vi "NMRglobal.vi"() -> ()   [LabVIEW 2013]
uses:
  <vilib>/Analysis/NI_AALBase.lvlib
panel:
  out "NMR Ave Graph":cluster{dbl, "Step Width (MHz)":dbl, dbl[][]}(graph)={224.69, "Step Width (MHz)"=0.002, [[-0.0025585333333335973, -0.0025785333333285033, -0.0021201333333384976, -0.0024833333333335096, -0.002168133333328727, -7.453333333811774e-05, -0.0018025333333334345, -0.003952133333328963, -0.0024233333333377447, -0.003016133333333376, -0.0035305333333292195, -0.00456653333333739, -0.004924133333333334, -0.007103333333329486, -0.0072041333333370495, -0.0031265333333333066, -0.0019705333333297687, -0.0005361333333367225, -0.001523333333333292, -0.0008321333333300675, 0.0001374666666635896, -0.00021453333333329298, 0.0004118666666696188, -0.00028333333333611444, -0.0004001333333333079, 0.004161466666669293, 0.001801466666664166, 0.0007198666666666612, 0.00171666666666895, -0.0009081333333355671, -0.0017545333333333839, -0.00012253333333140683, -0.0015121333333353152, -0.0021233333333334436, -0.0002561333333317787, -0.0012105333333350776, -0.0008865333333335181, -0.001584133333332165, -0.001903333333334855, -0.0022441333333336074, 9.346666666743345e-05, -0.0007905333333346475, 0.0017038666666662878, 0.005276666666667018, 0.007927866666665546, 0.008557466666666168, 0.012365466666666587, 0.02055186666666572, 0.028516666666666034, 0.03605986666666614, 0.041481466666665884, 0.04718146666666588, 0.045159866666665674, 0.04401666666666603, 0.03575186666666572, 0.028465466666665204, 0.02345746666666617, 0.020327866666665542, 0.017976666666664715, 0.014003866666666288, 0.013809466666665353, 0.014493466666664212, 0.014755866666666392, 0.008196666666665145, 0.009715866666667836, 0.008813466666666483, 0.009389466666664922, 0.008543866666668221, 0.0073766666666665575, 0.005687866666664685, 0.0066774666666685936, 0.005945466666666617, 0.0047918666666644325, 0.005516666666668951, 0.0014198666666666612, 0.0012014666666641661, 0.003161466666669293, 0.0032998666666666913, 0.00011666666666388487, -0.0009881333333303806, -0.0022145333333332923, 0.0013374666666635892, 0.00046786666666993155, 0.0008766666666667075, -0.0018361333333367235, -0.0004705333333297673, -0.0003265333333333061, -0.0020041333333370493, -0.001903333333329486, -0.0008241333333333347, -0.00236653333333739, -0.00313053333332922, 0.000583866666666625, 0.0019766666666622564, 0.002347866666671036, 0.004297466666666567, 0.005125466666661882, 0.004031866666671274, 0.006916666666666493, 0.0074798666666615, 0.006521466666671498], [-0.004151555000000268, -0.0032346549999951674, -0.0030565550000051585, -0.0030515550000001757, -0.003032154999995392, -0.0029464550000047837, -0.0028670550000001005, -0.002839254999995635, -0.0028472550000044083, -0.0028393550000000403, -0.0026902549999958864, -0.002623055000004056, -0.0025824550000000004, -0.002625554999996152, -0.002628855000003716, -0.002497254999999975, -0.002488654999996437, -0.002326755000003392, -0.002277254999999956, -0.0021894549999967312, -0.002116355000003079, -0.0020416549999999595, -0.002037954999997048, -0.0019417550000027821, -0.0018279549999999749, -0.0017424549999973742, -0.0016252550000024997, -0.0014985550000000051, -0.0013201549999977155, -0.0011361550000022333, -0.0010181550000000496, -0.0008573549999980733, -0.0006557550000019807, -0.00040805500000011004, -0.00021615499999844492, -2.1755000001744238e-05, 0.00028584499999981494, 0.0006856450000011681, 0.0012884449999984791, 0.0017766449999997254, 0.002533845000000767, 0.003499044999998682, 0.004639044999999614, 0.006053645000000351, 0.007976744999998881, 0.010652944999999504, 0.014275344999999917, 0.019335044999999062, 0.025848744999999354, 0.03369944499999943, 0.04110654499999926, 0.04502774499999923, 0.04310974499999907, 0.03670224499999938, 0.029105044999999042, 0.022443844999998505, 0.017336244999999504, 0.013608844999998863, 0.010775244999998053, 0.008735444999999623, 0.007194644999998683, 0.006035844999997543, 0.005142344999999731, 0.004461544999998471, 0.003983745000001169, 0.0036107449999998173, 0.0032414449999982517, 0.0030450450000015557, 0.0027286449999998916, 0.002523044999998015, 0.0023226450000019255, 0.0022273449999999527, 0.0021633449999977654, 0.002135445000002284, 0.002108244999999996, 0.0020771449999975, 0.0020462450000026285, 0.002019145000000028, 0.002081344999997216, 0.0020593450000029527, 0.002093945000000041, 0.002101344999996924, 0.002088845000003267, 0.0021361450000000398, 0.002182844999996609, 0.0021730450000035655, 0.002283045000000025, 0.0023518449999962803, 0.002430745000003849, 0.0024511449999999983, 0.0024622449999959417, 0.002504745000004117, 0.002607844999999958, 0.0026243449999955927, 0.002810745000004367, 0.0029247449999999075, 0.002920944999995217, 0.0030967450000046067, 0.0032808449999998245, 0.0032863449999948418, 0.003353545000004829]]}
  in  "COM Port #":refnum<visa-resource-name>="COM9"
  in  "GPIB Addr (28)":refnum<visa-resource-name>="GPIB0::28::INSTR"
  out "Pedestal (V)":dbl=-0.00048416666666591254 format="%_2g"
  in  "Open Global Panel":bool=TRUE
  out "Diff Sigma":dbl=0.003781704748572004 format="%#_13g"
  out "Peak center (MHz)":sgl=224.79416 format="%.3f"
  out "Peak width (MHz)":sgl=0.03243152 format="%.5f"
  out "Telnet error out":errorcluster
  out "Temperature (C)":dbl(graph)=26.5
  out "+3V supply":dbl=3.294 format="%_4g"
  out "Temp (C)":dbl=26.5 format="%_4g"
  out "RF OK":bool=TRUE
  out "Peak area (V-MHz)":sgl=0.00097212556 format="%.5f"
  out "NMR Graph + Fit":cluster{cluster{dbl, "Numeric":dbl}[]}[](graph)=[{[{224.69, "Numeric"=-0.0001132000000002584}, {224.692, "Numeric"=-0.00018210666666206715}, {224.694, "Numeric"=0.00022738666666173015}, {224.696, "Numeric"=-0.00018472000000018494}, {224.698, "Numeric"=8.157333333769484e-05}, {224.7, "Numeric"=0.0021262666666620957}, {224.702, "Numeric"=0.0003493599999998759}, {224.704, "Numeric"=-0.0018491466666625558}, {224.706, "Numeric"=-0.00036925333333754544}, {224.708, "Numeric"=-0.0010109600000000798}, {224.71, "Numeric"=-0.001574266666662826}, {224.712, "Numeric"=-0.002659173333337205}, {224.714, "Numeric"=-0.0030656800000000515}, {224.716, "Numeric"=-0.0052937866666631075}, {224.718, "Numeric"=-0.005443493333336879}, {224.72, "Numeric"=-0.0014148000000000387}, {224.722, "Numeric"=-0.000307706666663404}, {224.724, "Numeric"=0.001077786666663434}, {224.726, "Numeric"=4.167999999996172e-05}, {224.728, "Numeric"=0.000683973333336283}, {224.73, "Numeric"=0.0016046666666637318}, {224.732, "Numeric"=0.0012037599999999466}, {224.734, "Numeric"=0.0017812533333359552}, {224.736, "Numeric"=0.0010371466666640136}, {224.738, "Numeric"=0.0008714399999999173}, {224.74, "Numeric"=0.0053841333333356145}, {224.742, "Numeric"=0.00297522666666428}, {224.744, "Numeric"=0.0018447199999998723}, {224.74599999999998, "Numeric"=0.002792613333335953}, {224.748, "Numeric"=0.0001189066666645325}, {224.75, "Numeric"=-0.0007764000000001871}, {224.75199999999998, "Numeric"=0.0008066933333355817}, {224.754, "Numeric"=-0.0006318133333352298}, {224.756, "Numeric"=-0.0012919200000002613}, {224.75799999999998, "Numeric"=0.0005263733333351956}, {224.76, "Numeric"=-0.00047693333333500643}, {224.762, "Numeric"=-0.00020184000000034999}, {224.76399999999998, "Numeric"=-0.0009483466666652049}, {224.766, "Numeric"=-0.0013164533333347981}, {224.768, "Numeric"=-0.0017061600000004536}, {224.76999999999998, "Numeric"=0.0005825333333343793}, {224.772, "Numeric"=-0.0003503733333346048}, {224.774, "Numeric"=0.0020951199999994273}, {224.77599999999998, "Numeric"=0.005619013333333949}, {224.778, "Numeric"=0.008221306666665575}, {224.78, "Numeric"=0.008801999999999293}, {224.78199999999998, "Numeric"=0.012561093333333504}, {224.784, "Numeric"=0.020698586666665734}, {224.786, "Numeric"=0.028614479999999144}, {224.78799999999998, "Numeric"=0.036108773333333045}, {224.79, "Numeric"=0.041481466666665884}, {224.792, "Numeric"=0.04713255999999898}, {224.79399999999998, "Numeric"=0.04506205333333256}, {224.796, "Numeric"=0.043869946666666014}, {224.798, "Numeric"=0.0355562399999988}, {224.79999999999998, "Numeric"=0.028220933333332077}, {224.802, "Numeric"=0.023164026666666143}, {224.804, "Numeric"=0.019985519999998612}, {224.80599999999998, "Numeric"=0.017585413333331575}, {224.808, "Numeric"=0.013563706666666245}, {224.81, "Numeric"=0.013320399999998407}, {224.81199999999998, "Numeric"=0.013955493333331058}, {224.814, "Numeric"=0.014168986666666335}, {224.816, "Numeric"=0.0075608799999981845}, {224.81799999999998, "Numeric"=0.009031173333334667}, {224.82, "Numeric"=0.008079866666666411}, {224.822, "Numeric"=0.008606959999997948}, {224.82399999999998, "Numeric"=0.007712453333335039}, {224.826, "Numeric"=0.006496346666666472}, {224.828, "Numeric"=0.004758639999997696}, {224.82999999999998, "Numeric"=0.005699333333335397}, {224.832, "Numeric"=0.004918426666666517}, {224.834, "Numeric"=0.0037159199999974297}, {224.83599999999998, "Numeric"=0.00439181333333574}, {224.838, "Numeric"=0.00024610666666654733}, {224.83999999999997, "Numeric"=-2.120000000215591e-05}, {224.84199999999998, "Numeric"=0.0018898933333360679}, {224.844, "Numeric"=0.001979386666666563}, {224.84599999999998, "Numeric"=-0.0012527200000024513}, {224.84799999999998, "Numeric"=-0.00240642666666362}, {224.85, "Numeric"=-0.0036817333333334346}, {224.85199999999998, "Numeric"=-0.00017864000000276134}, {224.85399999999998, "Numeric"=-0.001097146666663322}, {224.856, "Numeric"=-0.0007372533333334491}, {224.85799999999998, "Numeric"=-0.0034989600000030884}, {224.85999999999999, "Numeric"=-0.002182266666663035}, {224.862, "Numeric"=-0.002087173333333477}, {224.86399999999998, "Numeric"=-0.0038136800000034285}, {224.86599999999999, "Numeric"=-0.003761786666662768}, {224.868, "Numeric"=-0.00273149333333352}, {224.86999999999998, "Numeric"=-0.004322800000003783}, {224.87199999999999, "Numeric"=-0.005135706666662516}, {224.874, "Numeric"=-0.0014702133333335744}, {224.87599999999998, "Numeric"=-0.00012632000000415127}, {224.878, "Numeric"=0.0001959733333377258}, {224.88, "Numeric"=0.0020966666666663537}, {224.88199999999998, "Numeric"=0.0028757599999954604}, {224.884, "Numeric"=0.0017332533333379494}, {224.886, "Numeric"=0.004569146666666265}, {224.88799999999998, "Numeric"=0.0050834399999950645}, {224.89, "Numeric"=0.004076133333338158}]}, {[{224.69, "Numeric"=6.623929819001648e-31}, {224.692, "Numeric"=8.258484058924611e-30}, {224.694, "Numeric"=9.8048498042907e-29}, {224.696, "Numeric"=1.1085047385032389e-27}, {224.698, "Numeric"=1.1934113410424357e-26}, {224.7, "Numeric"=1.2234853274178262e-25}, {224.702, "Numeric"=1.194437331048164e-24}, {224.704, "Numeric"=1.1104115474083053e-23}, {224.706, "Numeric"=9.830159591286655e-23}, {224.708, "Numeric"=8.286920373635448e-22}, {224.71, "Numeric"=6.652452177829644e-21}, {224.712, "Numeric"=5.0854144731305415e-20}, {224.714, "Numeric"=3.7019192930940836e-19}, {224.716, "Numeric"=2.566158847051204e-18}, {224.718, "Numeric"=1.6939325907935165e-17}, {224.72, "Numeric"=1.0647918288367481e-16}, {224.722, "Numeric"=6.373665888513903e-16}, {224.724, "Numeric"=3.633037460074899e-15}, {224.726, "Numeric"=1.9719979363193455e-14}, {224.728, "Numeric"=1.0192929830304985e-13}, {224.73, "Numeric"=5.01704054672824e-13}, {224.732, "Numeric"=2.3515389979905417e-12}, {224.734, "Numeric"=1.0495732612802684e-11}, {224.736, "Numeric"=4.46097027043166e-11}, {224.738, "Numeric"=1.8055183134255389e-10}, {224.74, "Numeric"=6.958737670807953e-10}, {224.742, "Numeric"=2.553965521259862e-09}, {224.744, "Numeric"=8.925973500679592e-09}, {224.74599999999998, "Numeric"=2.9706545690318888e-08}, {224.748, "Numeric"=9.414661590474801e-08}, {224.75, "Numeric"=2.84127500941467e-07}, {224.75199999999998, "Numeric"=8.165406818902004e-07}, {224.754, "Numeric"=2.234592726911031e-06}, {224.756, "Numeric"=5.823377347801665e-06}, {224.75799999999998, "Numeric"=1.4451318831929812e-05}, {224.76, "Numeric"=3.4150418553862735e-05}, {224.762, "Numeric"=7.684941697660145e-05}, {224.76399999999998, "Numeric"=0.00016468009973493478}, {224.766, "Numeric"=0.00033604517473984904}, {224.768, "Numeric"=0.0006529955238538497}, {224.76999999999998, "Numeric"=0.0012083110382988984}, {224.772, "Numeric"=0.0021291353944581197}, {224.774, "Numeric"=0.0035725952339053053}, {224.77599999999998, "Numeric"=0.005708478207812643}, {224.778, "Numeric"=0.00868586106957128}, {224.78, "Numeric"=0.012585237269448659}, {224.78199999999998, "Numeric"=0.017364646035845876}, {224.784, "Numeric"=0.022815314535005283}, {224.786, "Numeric"=0.02854585029721257}, {224.78799999999998, "Numeric"=0.034010694904734115}, {224.79, "Numeric"=0.038587267454119216}, {224.792, "Numeric"=0.04168967821984403}, {224.79399999999998, "Numeric"=0.04289128513101013}, {224.796, "Numeric"=0.042020921594759224}, {224.798, "Numeric"=0.039202890109446005}, {224.79999999999998, "Numeric"=0.03482784439654041}, {224.802, "Numeric"=0.02946395915701044}, {224.804, "Numeric"=0.02373622282600602}, {224.80599999999998, "Numeric"=0.018209084651893668}, {224.808, "Numeric"=0.013302112534378378}, {224.81, "Numeric"=0.009253565819657653}, {224.81199999999998, "Numeric"=0.006129903212458004}, {224.814, "Numeric"=0.0038668214081623727}, {224.816, "Numeric"=0.0023227935396983946}, {224.81799999999998, "Numeric"=0.0013286882753878616}, {224.82, "Numeric"=0.0007237550283915916}, {224.822, "Numeric"=0.00037541885735998127}, {224.82399999999998, "Numeric"=0.00018543707619032908}, {224.826, "Numeric"=8.722340906752696e-05}, {224.828, "Numeric"=3.906839235205798e-05}, {224.82999999999998, "Numeric"=1.6663799152561437e-05}, {224.832, "Numeric"=6.768282891409274e-06}, {224.834, "Numeric"=2.617815172957578e-06}, {224.83599999999998, "Numeric"=9.641740903748032e-07}, {224.838, "Numeric"=3.381644354052067e-07}, {224.83999999999997, "Numeric"=1.1294224172854167e-07}, {224.84199999999998, "Numeric"=3.592037600537461e-08}, {224.844, "Numeric"=1.0878808771350877e-08}, {224.84599999999998, "Numeric"=3.1374571962168593e-09}, {224.84799999999998, "Numeric"=8.616487739674512e-10}, {224.85, "Numeric"=2.2534023213654733e-10}, {224.85199999999998, "Numeric"=5.6118130992194455e-11}, {224.85399999999998, "Numeric"=1.3308332952595468e-11}, {224.856, "Numeric"=3.0053850032780303e-12}, {224.85799999999998, "Numeric"=6.462976404817905e-13}, {224.85999999999999, "Numeric"=1.3234910961652932e-13}, {224.862, "Numeric"=2.5808661142638485e-14}, {224.86399999999998, "Numeric"=4.792541975037948e-15}, {224.86599999999999, "Numeric"=8.474661749212857e-16}, {224.868, "Numeric"=1.427035638060203e-16}, {224.86999999999998, "Numeric"=2.288248904814317e-17}, {224.87199999999999, "Numeric"=3.494038655156257e-18}, {224.874, "Numeric"=5.08051976932488e-19}, {224.87599999999998, "Numeric"=7.034683845409073e-20}, {224.878, "Numeric"=9.275493395705102e-21}, {224.88, "Numeric"=1.1646232479308655e-21}, {224.88199999999998, "Numeric"=1.3924829552296147e-22}, {224.884, "Numeric"=1.5854418531574358e-23}, {224.886, "Numeric"=1.7189638662592754e-24}, {224.88799999999998, "Numeric"=1.7747581315264437e-25}, {224.89, "Numeric"=1.7448881764805936e-26}]}]
  out "Pedestal Offset":dbl(graph)=-0.00048416666666591254
  out "Pedestal Difference":dbl(graph)=0.003423466666666674
  out "# Good Spectra":i32=991
  out "Pedestal OK":bool=TRUE
  out "Sweep #":i32=1000
  out "1st Sweep":bool
  out "ADC volts OK":bool=TRUE
  out "Peak Height Distribution":cluster{"Y":dbl[], "Y":dbl[]}[](graph)=[{"Y"=[0.03404756086642266, 0.034186998232694187, 0.03432643559896571, 0.03446587296523724, 0.034605310331508765, 0.03474474769778029, 0.03488418506405182, 0.035023622430323344, 0.03516305979659487, 0.035302497162866396, 0.035441934529137915, 0.03558137189540944, 0.03572080926168097, 0.035860246627952494, 0.03599968399422402, 0.036139121360495546, 0.03627855872676707, 0.0364179960930386, 0.036557433459310125, 0.03669687082558165, 0.03683630819185317, 0.0369757455581247, 0.03711518292439622, 0.03725462029066775, 0.037394057656939275, 0.0375334950232108, 0.03767293238948233, 0.037812369755753854, 0.03795180712202538, 0.038091244488296906, 0.038230681854568425, 0.03837011922083995, 0.03850955658711148, 0.038648993953383004, 0.03878843131965453, 0.038927868685926056, 0.03906730605219758, 0.03920674341846911, 0.039346180784740635, 0.03948561815101216, 0.03962505551728368, 0.03976449288355521, 0.03990393024982673, 0.04004336761609826, 0.040182804982369785, 0.04032224234864131, 0.04046167971491284, 0.040601117081184364, 0.04074055444745589, 0.040879991813727416, 0.041019429179998936, 0.04115886654627046, 0.04129830391254199, 0.041437741278813514, 0.04157717864508504, 0.041716616011356566, 0.04185605337762809, 0.04199549074389962, 0.042134928110171145, 0.04227436547644267, 0.04241380284271419, 0.04255324020898572, 0.04269267757525724, 0.04283211494152877, 0.042971552307800295, 0.04311098967407182, 0.04325042704034335, 0.043389864406614874, 0.0435293017728864, 0.043668739139157926, 0.043808176505429446, 0.04394761387170097, 0.0440870512379725, 0.044226488604244024, 0.04436592597051555, 0.04450536333678708, 0.0446448007030586, 0.04478423806933013, 0.044923675435601655, 0.04506311280187318, 0.0452025501681447, 0.04534198753441623, 0.04548142490068775, 0.04562086226695928, 0.045760299633230805, 0.04589973699950233, 0.04603917436577386, 0.046178611732045384, 0.04631804909831691, 0.046457486464588436, 0.046596923830859956, 0.04673636119713148, 0.04687579856340301, 0.047015235929674534, 0.04715467329594606, 0.04729411066221759, 0.04743354802848911, 0.04757298539476064, 0.047712422761032165, 0.04785186012730369], "Y"=[1.0, 0.0, 0.0, 0.0, 1.0, 0.0, 1.0, 2.0, 4.0, 2.0, 4.0, 4.0, 3.0, 3.0, 6.0, 5.0, 6.0, 4.0, 2.0, 6.0, 4.0, 7.0, 6.0, 8.0, 8.0, 8.0, 10.0, 11.0, 15.0, 12.0, 19.0, 7.0, 10.0, 18.0, 8.0, 15.0, 14.0, 25.0, 17.0, 15.0, 11.0, 16.0, 23.0, 19.0, 13.0, 19.0, 25.0, 24.0, 21.0, 17.0, 23.0, 21.0, 16.0, 23.0, 14.0, 17.0, 16.0, 21.0, 19.0, 25.0, 12.0, 16.0, 17.0, 14.0, 9.0, 17.0, 18.0, 12.0, 12.0, 16.0, 16.0, 8.0, 9.0, 14.0, 7.0, 8.0, 9.0, 13.0, 13.0, 6.0, 5.0, 6.0, 9.0, 4.0, 6.0, 5.0, 6.0, 3.0, 5.0, 4.0, 4.0, 2.0, 3.0, 1.0, 4.0, 0.0, 0.0, 1.0, 2.0, 1.0]}]
  out "S/N":dbl=15.348964814234717 format="%_3g"
  out "Peak mean (V)":dbl=0.04111339610790677 format="%_4g"
  out "Peak Height":dbl(graph)=0.04289815043584681
  out "Voltage Array":sgl[](array[numeric])=[0.0245, 0.0234, 0.0228, 0.0214, 0.0207, 0.0218, 0.0191, 0.016, 0.0166, 0.0151, 0.0137, 0.0118, 0.0106, 0.0076, 0.0067, 0.01, 0.0104, 0.0111, 0.0094, 0.0094, 0.0097, 0.0087, 0.0087, 0.0074, 0.0067, 0.0107, 0.0078, 0.0062, 0.0067, 0.0036, 0.0023, 0.0035, 0.0017, 0.0007, 0.0022, 0.0009, 0.0009, -0.0001, -0.0007, -0.0013, 0.0008, -0.0003, 0.002, 0.0054, 0.0079, 0.0084, 0.0121, 0.0202, 0.0281, 0.0356, 0.041, 0.0467, 0.0447, 0.0436, 0.0354, 0.0282, 0.0233, 0.0203, 0.0181, 0.0143, 0.0143, 0.0152, 0.0157, 0.0094, 0.0112, 0.0106, 0.0115, 0.011, 0.0102, 0.0089, 0.0103, 0.01, 0.0093, 0.0105, 0.0069, 0.0072, 0.0097, 0.0104, 0.0078, 0.0073, 0.0067, 0.0109, 0.0107, 0.0118, 0.0098, 0.0119, 0.0128, 0.0119, 0.0128, 0.0147, 0.014, 0.0141, 0.0187, 0.021, 0.0223, 0.0252, 0.027, 0.0269, 0.0308, 0.0324, 0.0325] format="%.4f"
  out "Pedestal Diff (V)":sgl=0.0034234666 format="%.3f"
  out "Peak amp (V)":sgl=0.042898152 format="%.3f"
  out "SMT error out":errorcluster
  out "Sample RMS (V)":dbl=0.00182970297029703 format="%.4f"
  in  "Sweep Mode":u16(ring)=3 items=["Off", "Single", "Auto", "Step"]
  # "E1039 NMR Panel"
  # "Results"
  # "A\nv\ne\nr\na\ng\ne"
  # "S\nw\ne\ne\np"
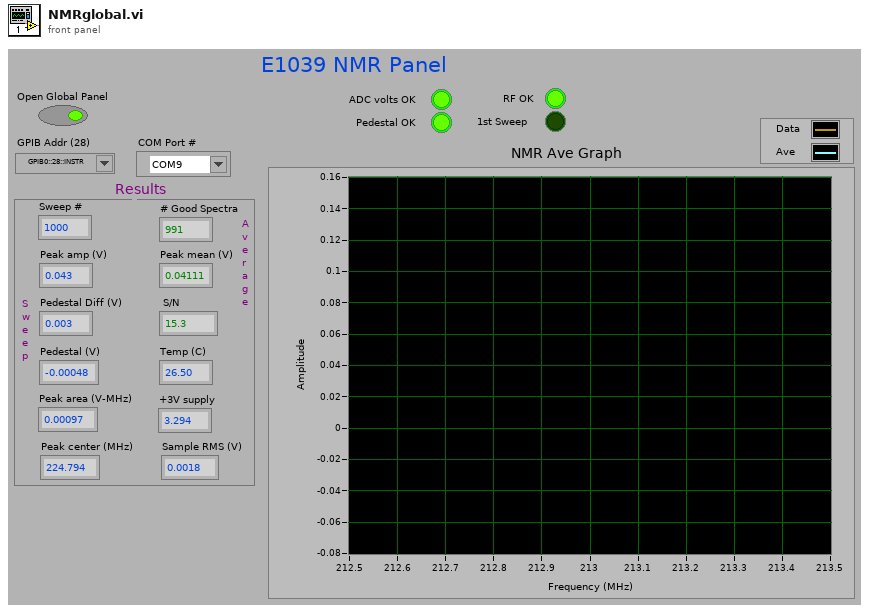
[diagram p1: front panel]
types:
  T1 = enum32{"Invalid", "Standard", "Closed", "Hidden", "Minimized", "Maximized"}
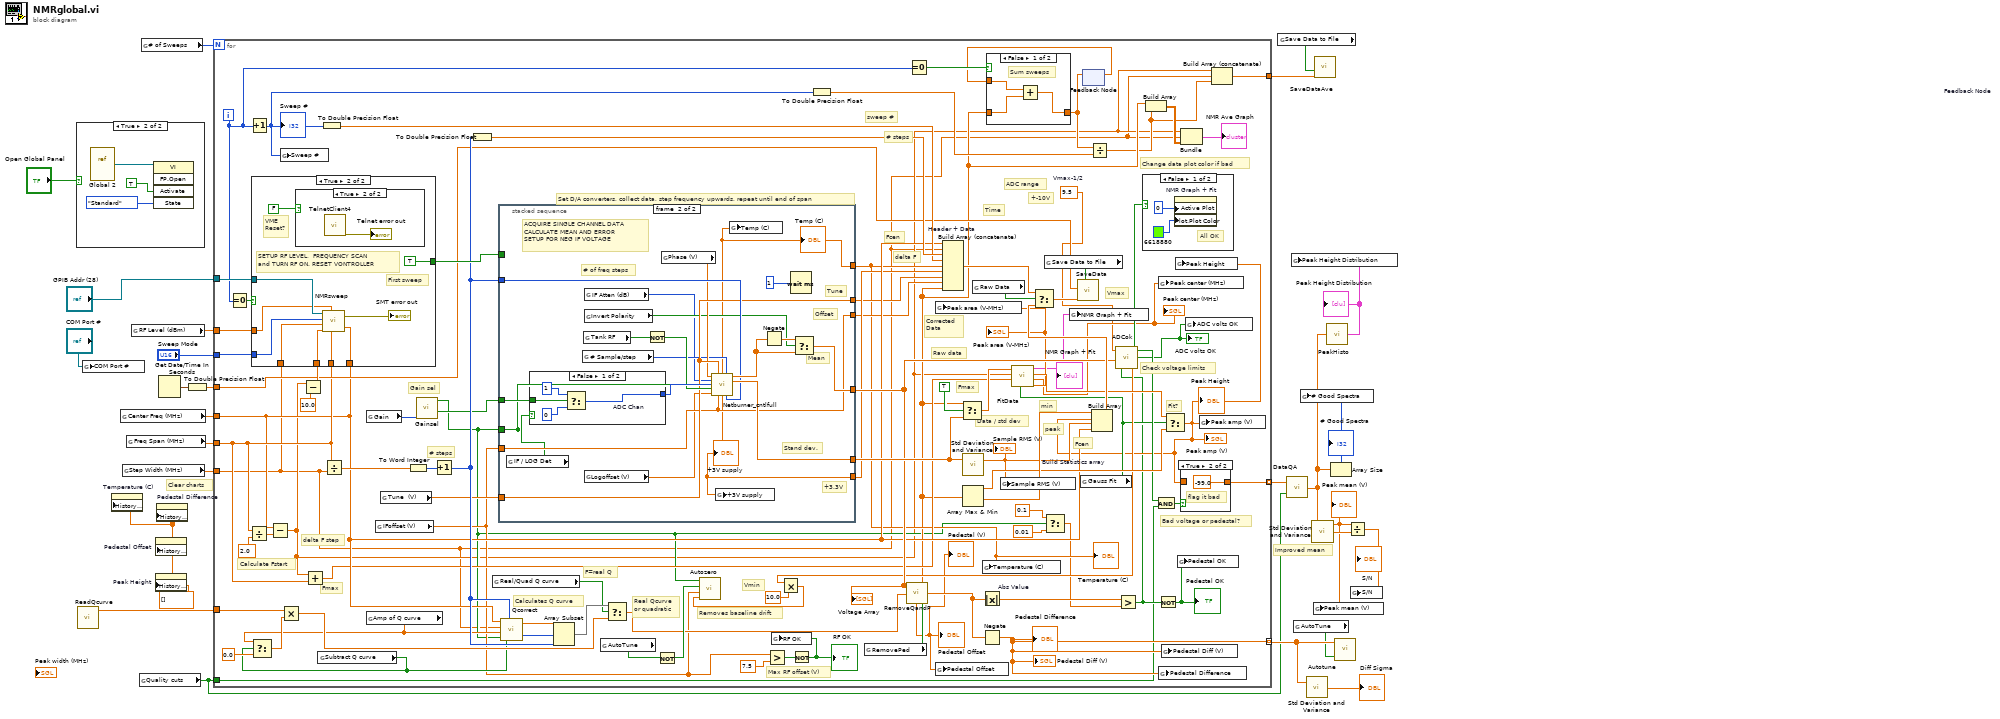
[diagram p0: block diagram]
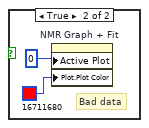
[diagram p4: hidden frame]
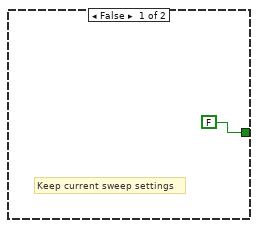
[diagram p6: hidden frame]
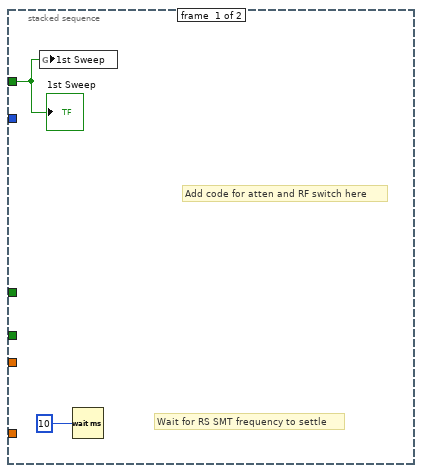
[diagram p8: hidden frame]
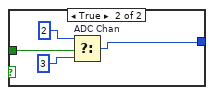
[diagram p9: hidden frame]
diagram:
  w22 = dbl[] []
  # "Clear charts"
  # "Improved mean"
  n1 = case shown="True" "Open Global Panel" {
    frame False {
    }
    frame True {
      n2 = vi-ref "Global 2.vi"() -> (w29:refnum<vi>)
      n3 = invoke class="VI" method="FP.Open"(reference=w29, "Activate"=TRUE, "State"=T1."Standard") -> ()  [unwired: 2 in, 5 out]
    }
  }
  n4 = call "ReadQcurve.vi"() -> ("Array"=w1:dbl[])  [unwired: 2 in]
  n5 = global write "Global 2.vi" "COM Port #"("COM Port #") -> ()
  n6 = property on="Temperature (C)" class="WFChart (strict)"("History Data"=w22) -> ()  [unwired: 2 in, 2 out]
  n7 = global read "Global 2.vi" "Center Freq (MHz)"() -> (w16:dbl)
  n8 = global read "Global 2.vi" "Step Width (MHz)"() -> (w14:dbl)
  n9 = global read "Global 2.vi" "Freq Span (MHz)"() -> (w15:dbl)
  n10 = global read "Global 2.vi" "RF Level (dBm)"() -> (w17:dbl)
  n11 = global read "Global 2.vi" "Quality cuts"() -> (w13:bool)
  n12 = global read "Global 2.vi" "# of Sweeps"() -> (w18:i32)
  n13 = property on="Peak Height" class="WFChart (strict)"("History Data"=w22) -> ()  [unwired: 2 in, 2 out]
  n14 = property on="Pedestal Offset" class="WFChart (strict)"("History Data"=w22) -> ()  [unwired: 2 in, 2 out]
  n15 = property on="Pedestal Difference" class="WFChart (strict)"("History Data"=w22) -> ()  [unwired: 2 in, 2 out]
  n16 = Get Date/Time In Seconds() -> (seconds since 1Jan1904=w23:timestamp)
  n17 = To Double Precision Float(number=w23) -> (double precision float=w2:dbl)
  n18 = for {
    N: w18 -> [_]
    tunnel: [w108] -> w26 mode=indexing
    tunnel: w13 -> [w48]
    tunnel: [w55] -> w20 mode=indexing
    tunnel: w16 -> [w90]
    tunnel: w15 -> [w94]
    tunnel: w14 -> [w31]
    tunnel: "Sweep Mode" -> [w100]
    tunnel: "GPIB Addr (28)" -> [w99]
    tunnel: w17 -> [w98]
    tunnel: w2 -> [w95]
    tunnel: w1 -> [w82]
    tunnel: [w30] -> w4
    i -> [w44]
    w41 = 9.5  # Vmax-1/2
    # "Gain sel"
    # "F=real Q"
    # "Real Qcurve\nor quadratic"
    # "+-10V"
    # "Vmax"
    # "Change data plot color if bad"
    # "Max RF offset (V)"
    # "Fmax"
    # "Fit?"
    # "Fmax"
    # "Time"
    # "Vmin"
    # "min"
    # "peak"
    # "Raw data"
    # "Corrected\nData"
    # "Fcen"
    # "delta F"
    # "# steps"
    # "ADC range"
    # "sweep #"
    # "Fcen"
    # "Set D/A converters, collect data, step frequency upwards, repeat until end of span"
    # "Calculates Q curve"
    # "Removes baseline drift"
    # "Bad voltage or pedestal?"
    # "Check voltage limits"
    # "Data / std dev"
    # "# steps"
    # "Calculate Fstart"
    # "delta F step"
    n19 = Equal To 0?(x=w44) -> (x = 0?=w110:bool)
    n20 = Divide(x=w94, y=sgl 2.0) -> (x/y=w120:dbl)
    n21 = Increment(x=w44) -> (x+1=w46:i32)
    "Sweep #" <- w46
    n22 = Subtract(x=w90, y=w120) -> (x-y=w32:dbl)
    n23 = global write "Global 2.vi" "Sweep #"(w46) -> ()
    n24 = Subtract(x=w32, y=10.0) -> (x-y=w118:dbl)
    n25 = case shown="True" w110 {
      tunnel: w118 -> [_ w143]
      tunnel: w31 -> [_ w141]
      tunnel: w90 -> [_ w140]
      tunnel: w94 -> [_ w142]
      tunnel: [FALSE TRUE] -> w109
      tunnel: w100 -> [_ w137]
      tunnel: w99 -> [_ w136]
      tunnel: w98 -> [_ w135]
      frame False {
        # "Keep current sweep settings"
      }
      frame True {
        # "VME\nReset?"
        # "First sweep"
        # "SETUP RF LEVEL,  FREQUENCY SCAN\nand TURN RF ON. RESET VONTROLLER"
        n26 = case shown="True" FALSE {
          frame False {
          }
          frame True {
            n27 = call "TelnetClient4.vi"() -> ("Telnet error"=→"Telnet error out":errorcluster)  [unwired: 4 in, 3 out]
          }
        }
        n28 = call "NMRsweep.vi"("Center Freq (MHz)"=w140, "Freq Span (MHz)"=w142, "RF Level (dBm)"=w135, "Foffset (MHz)"=w143, "Step Width (MHz)"=w141, "Sweep Mode"=w137, "GPIB Addr (28)"=w136) -> ("error out"=→"SMT error out":errorcluster)
      }
    }
    n29 = Add(x=w32, y=w94) -> (x+y=w87:dbl)
    n30 = global read "Global 2.vi" "Subtract Q curve"() -> (w70:bool)
    n31 = To Double Precision Float(number=w46) -> (double precision float=w101:dbl)
    n32 = Divide(x=w94, y=w31) -> (x/y=w122:dbl)
    n33 = global read "Global 2.vi" "Amp of Q curve"() -> (w71:dbl)
    n34 = Select(t=w71, s=w70, f=0.0) -> (s? t:f=w79:dbl)
    n35 = Multiply(x=w82, y=w79) -> (x*y=w81:dbl[])
    n36 = global read "Global 2.vi" "Gain"() -> (w35:enum16{"LOW", "HI", "MAX"})
    n37 = global read "Global 2.vi" "IFoffset (V)"() -> (w52:dbl)
    n38 = global read "Global 2.vi" "Tune  (V)"() -> (w72:dbl)
    n39 = To Word Integer(number=w122) -> (16bit integer=w119:i16)
    n40 = call "Gainsel.vi"("Gain"=w35) -> ("LO"=w36:bool, "MAX"=w34:bool)  [unwired: 1 out]
    n41 = Increment(x=w119) -> (x+1=w103:i16)
    n42 = To Double Precision Float(number=w103) -> (double precision float=w102:dbl)
    n43 = global read "Global 2.vi" "Real/Quad Q curve"() -> (w69:bool)
    n44 = stacked-sequence {
      tunnel: [_ w162] -> w113
      tunnel: [_ w166] -> w97
      tunnel: w103 -> [_ w160]
      tunnel: w52 -> [_ w157]
      tunnel: w36 -> [_ w164]
      tunnel: w109 -> [w145 _]
      tunnel: w72 -> [_ w158]
      tunnel: [_ w148] -> w54
      tunnel: [_ w147] -> w78
      tunnel: [_ w158] -> w77
      tunnel: [_ w157] -> w76
      tunnel: [_ w156] -> _
      tunnel: w34 -> [_ w156]
      frame #0 {
        # "Add code for atten and RF switch here"
        # "Wait for RS SMT frequency to settle"
        n45 = global write "Global 2.vi" "1st Sweep"(w145) -> ()
        n46 = Wait (ms)(milliseconds to wait=10) -> ()  [unwired: 1 out]
        "1st Sweep" <- w145
      }
      frame #1 {
        # "+3.3V"
        # "Offset"
        # "Tune"
        # "Stand dev."
        # "Mean"
        # "ACQUIRE SINGLE CHANNEL DATA\nCALCULATE MEAN AND ERROR\nSETUP FOR NEG IF VOLTAGE"
        # "# of freq steps"
        n47 = global read "Global 2.vi" "IF / LOG Det"() -> (w153:bool)
        n48 = case shown="False" w153 {
          tunnel: w164 -> [w171 w172]
          tunnel: [w168 w173] -> w161
          frame False {
            n49 = Select "ADC Chan"(t=1, s=w171, f=0) -> (s? t:f=w168:i32)
          }
          frame True {
            n50 = Select "ADC Chan"(t=2, s=w172, f=3) -> (s? t:f=w173:i32)
          }
        }
        n51 = global read "Global 2.vi" "# Sample/step"() -> (w150:i32)
        n52 = global read "Global 2.vi" "Tank RF"() -> (w152:bool)
        n53 = global read "Global 2.vi" "Invert Polarity"() -> (w151:bool)
        n54 = global read "Global 2.vi" "Logoffset (V)"() -> (w154:dbl)
        n55 = global read "Global 2.vi" "IF Atten (dB)"() -> (w149:i8)
        n56 = Not(x=w152) -> (.not. x?=w159:bool)
        n57 = global read "Global 2.vi" "Phase (V)"() -> (w155:dbl)
        n58 = call "Netburner_cntlfull.vi"("Phase Volt"=w155, "Tune Volt"=w158, "# Data"=w150, "IF Atten (dB)"=w149, "NMR ADC"=w161, "Hi Gain"=w156, "Tank RF"=w159, "LogOff Volt"=w154, "IFOff Volt"=w157, "# f steps"=w160) -> ("Temp (C)"=w148:dbl, "ADC value"=w163:dbl[], "ADC error"=w162:dbl[], "Volts"=w147:dbl)  [unwired: 2 out]
        "Temp (C)" <- w148
        "+3V supply" <- w147
        n59 = global write "Global 2.vi" "+3V supply"(w147) -> ()
        n60 = global write "Global 2.vi" "Temp (C)"(w148) -> ()
        n61 = Negate(x=w163) -> (-x=w165:dbl[])
        n62 = Wait (ms)(milliseconds to wait=1) -> ()  [unwired: 1 out]
        n63 = Select(t=w165, s=w151, f=w163) -> (s? t:f=w166:dbl[])
      }
    }
    "Voltage Array" <- w97
    "Temperature (C)" <- w54
    n64 = call "Qcorrect.vi"("Subtract Q curve"=w70, "Nstep"=w103, "Max Gain"=w34, "Amp of Q curve"=w71, "Step Width (MHz)"=w31, "Center Freq (MHz)"=w90) -> ("Start"=w114:i32, "Array"=w115:dbl[])
    n65 = Array Subset "Array Subset"(array=w115, index=w114, length=w103) -> (w84:dbl[])
    n66 = global read "Global 2.vi" "AutoTune"() -> (w67:bool)
    n67 = Select(t=w84, s=w69, f=w81) -> (s? t:f=w83:dbl[])
    n68 = Not(x=w67) -> (.not. x?=w85:bool)
    n69 = Greater?(x=w52, y=7.5) -> (0:w91:bool)
    n70 = Not(x=w91) -> (.not. x?=w61:bool)
    "RF OK" <- w61
    n71 = global write "Global 2.vi" "RF OK"(w61) -> ()
    n72 = To Double Precision Float(number=w46) -> (double precision float=w39:dbl)
    n73 = global read "Global 2.vi" "RemovePed"() -> (w68:bool)
    n74 = call "RemoveQandP.vi"("Subtract Ped?"=w68, "Qcurve"=w83, "Raw data"=w97) -> ("Ped L-R"=w105:dbl, "Corrected data"=w38:dbl[], "Ped Offfset"=w53:dbl)
    "Pedestal Offset" <- w53
    "Pedestal (V)" <- w53
    n75 = Equal To 0?(x=w44) -> (x = 0?=w45:bool)
    n76 = global write "Global 2.vi" "Pedestal Offset"(w53) -> ()
    n77 = Build Array (concatenate) "Header + Data"(w90, w31, w102, w101, w54, w78, w77, w76, w38) -> (w104:dbl[])
    n78 = Select(t=w38, s=TRUE, f=w113) -> (s? t:f=w88:dbl[])
    n79 = call <vilib>:"Std Deviation and Variance.vi"("X"=w113) -> ("mean"=w59:dbl)  [unwired: 1 in, 2 out]
    "Sample RMS (V)" <- w59
    n80 = Array Max & Min(array=w38) -> (max value=w93:dbl, min value=w112:dbl)  [unwired: 2 out]
    n81 = global read "Global 2.vi" "Raw Data"() -> (w65:bool)
    n82 = Absolute Value "Abs Value"(x=w105) -> (abs(x)=w106:dbl)
    n83 = Negate(x=w105) -> (-x=w55:dbl)
    "Pedestal Diff (V)" <- w55
    "Pedestal Difference" <- w55
    n84 = global write "Global 2.vi" "Temperature (C)"(w54) -> ()
    n85 = global write "Global 2.vi" "Sample RMS (V)"(w59) -> ()
    n86 = global read "Global 2.vi" "Save Data to File"() -> (w66:bool)
    n87 = Select(t=0.1, s=w34, f=0.01) -> (s? t:f=w47:dbl)
    n88 = global read "Global 2.vi" "Gauss Fit"() -> (w64:bool)
    n89 = call "FitData.vi"("Fit?"=w64, "Fmax"=w87, "Fmin"=w32, "Yarray"=w88) -> ("Peak Area (V-MHz)"=w60:dbl, "Center Freq (MHz)"=w58:dbl, "Amplitude (V)"=w89:dbl, "NMR Graph + Fit"=w56:cluster{cluster{dbl, "Numeric":dbl}[]}[])  [unwired: 1 out]
    "NMR Graph + Fit" <- w56
    "Peak area (V-MHz)" <- w60
    "Peak center (MHz)" <- w58
    n90 = global write "Global 2.vi" "Peak area (V-MHz)"(w60) -> ()
    n91 = global write "Global 2.vi" "NMR Graph + Fit"(w56) -> ()
    n92 = feedback #1 "Feedback Node"() -> (w43:dbl[])  [unwired: 1 in]
    n93 = case shown="False" w45 {
      tunnel: w38 -> [w124 w126]
      tunnel: [w123 w126] -> w40
      tunnel: w43 -> [w125 _]
      frame False {
        # "Sum sweeps"
        n94 = Add(x=w125, y=w124) -> (x+y=w123:dbl[])
      }
      frame True {
        # "Initialize"
      }
    }
    n95 = feedback-in #1(w40) -> ()
    n96 = Divide(x=w40, y=w39) -> (x/y=w33:dbl[])
    n97 = Greater?(x=w106, y=w47) -> (0:w49:bool)
    n98 = call "ADCok.vi"("PedOK"=w49, "Array"=w97, "Vmax-1/2"=w41) -> ("Vmin"=w75:dbl, "ADC voltages OK"=w63:bool, "Allok"=w86:bool)
    "ADC volts OK" <- w63
    n99 = Multiply(x=w75, y=10.0) -> (x*y=w73:dbl)
    n100 = call "Autozero.vi"("Vmin (V)"=w73, "IFoffset (V)"=w52, "Enable"=w85, "Max Gain"=w34) -> ()
    n101 = case shown="False" w86 {
      frame False {
        # "All OK"
        n102 = property on="NMR Graph + Fit" class="XYGraph (strict)"("Active Plot"=0, "Plot.Plot Color"=u32 6618880) -> ()  [unwired: 2 in, 2 out]
      }
      frame True {
        # "Bad data"
        n103 = property on="NMR Graph + Fit" class="XYGraph (strict)"("Active Plot"=0, "Plot.Plot Color"=u32 16711680) -> ()  [unwired: 2 in, 2 out]
      }
    }
    n104 = Build Array "Build Array"(w38, w33) -> (w37:dbl[][])
    n105 = And(x=w86, y=w48) -> (x .and. y?=w107:bool)
    n106 = Not(x=w49) -> (.not. x?=w62:bool)
    "Pedestal OK" <- w62
    n107 = global write "Global 2.vi" "Peak center (MHz)"(w58) -> ()
    n108 = global write "Global 2.vi" "Pedestal Difference"(w55) -> ()
    n109 = global write "Global 2.vi" "Pedestal Diff (V)"(w55) -> ()
    n110 = Select(t=w89, s=w64, f=w93) -> (s? t:f=w57:dbl)
    "Peak amp (V)" <- w57
    "Peak Height" <- w57
    n111 = Build Array "Build Statistics array"(w112, w57, w59, w90) -> (w117:dbl[])
    n112 = Select(t=w104, s=w65, f=w117) -> (s? t:f=w96:dbl[])
    n113 = call "SaveData.vi"("Array"=w96, "Save Data to File"=w66, "Ext time (sec)"=w95) -> ()  [unwired: 1 out]
    n114 = global write "Global 2.vi" "Peak Height"(w57) -> ()
    n115 = global write "Global 2.vi" "Pedestal OK"(w62) -> ()
    n116 = Bundle(w32, "Step Width (MHz)"=w31, w37) -> (→"NMR Ave Graph":cluster{dbl, "Step Width (MHz)":dbl, dbl[][]})  [unwired: 1 in]
    n117 = case shown="True" w107 {
      tunnel: [w131 -99.0] -> w108
      tunnel: w57 -> [w131 _]
      frame False {
        # "Data OK"
      }
      frame True {
        # "flag it bad"
      }
    }
    n118 = global write "Global 2.vi" "ADC volts OK"(w63) -> ()
    n119 = global write "Global 2.vi" "Peak amp (V)"(w57) -> ()
    n120 = Build Array (concatenate) "Build Array"(w32, w31, w33) -> (w30:dbl[])
  }
  n121 = global read "Global 2.vi" "Save Data to File"() -> (w3:bool)
  n122 = call "DataQA.vi"("Quality cuts"=w13, "Data In"=w26) -> ("Data Out"=w25:dbl[])
  n123 = global read "Global 2.vi" "AutoTune"() -> (w12:bool)
  n124 = call <vilib>:"Std Deviation and Variance.vi"("X"=w20) -> ("standard deviation"=→"Diff Sigma":dbl)  [unwired: 1 in, 2 out]
  n125 = call <vilib>:"Std Deviation and Variance.vi"("X"=w25) -> ("mean"=w10:dbl, "standard deviation"=w21:dbl)  [unwired: 1 in, 1 out]
  "Peak mean (V)" <- w10
  n126 = global write "Global 2.vi" "Peak mean (V)"(w10) -> ()
  n127 = call "SaveDataAve.vi"("Array"=w4, "Save Data to File"=w3) -> ()  [unwired: 1 in, 1 out]
  n128 = call "PeakHisto.vi"("Data Out"=w25) -> ("XY Graph"=w8:cluster{"Y":dbl[], "Y":dbl[]}[])
  "Peak Height Distribution" <- w8
  n129 = global write "Global 2.vi" "Peak Height Distribution"(w8) -> ()
  n130 = Array Size(array=w25) -> (size(s)=w9:i32)
  "# Good Spectra" <- w9
  n131 = global write "Global 2.vi" "# Good Spectra"(w9) -> ()
  n132 = call "Autotune.vi"("Adjust Tune"=w12, "Pedestal Diff"=w20) -> ()  [unwired: 1 in, 1 out]
  n133 = Divide(x=w10, y=w21) -> (x/y=w11:dbl)
  "S/N" <- w11
  n134 = global write "Global 2.vi" "S/N"(w11) -> ()
